vi "medicaoIXV.vi"() -> ()   [LabVIEW 2012]
uses:
  <vilib>/Utility/file.llb/Write To Spreadsheet File (string).vi
  <vilib>/Utility/file.llb/Write To Spreadsheet File (DBL).vi
  <instrlib>/Agilent 6XXX Series/Agilent 6XXX Series.lvlib
panel:
  out "array":dbl[][](array[numeric])
  in  "Tab Control":enum32{"Entrada de dados", "Saída de dados"}(tab)
  out "ON/OFF":bool
  in  "Pontos":dbl
  in  "Tensão máxima":dbl
  in  "Nome da célula":string
  in  "Local":path
  in  "Delay(s)":dbl
  in  "Start":bool
  out "IXV":cluster{"Y":dbl[], "Y":dbl[]}[](graph)
  out "output voltage":dbl
  out "Tensao Atual":dbl
  out "Corrente Atual":dbl
  out "Ponto Atual":i32
  out "TABELA DE DADOS\nTensão(fonte)     Tensão                  Corrente            Pontos":dbl[][](array[numeric]) caption="all rows" format="%0.3f"
  in  "CorrenteGraph":dbl
  in  "error in (no error)":errorcluster
  out "error out":errorcluster
  in  "TensaoGraph":dbl
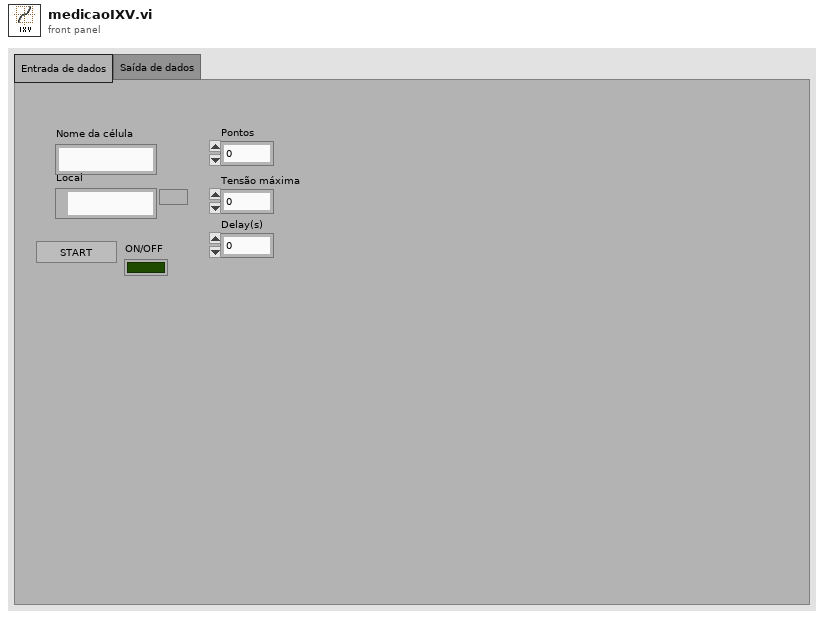
[diagram p1: front panel]
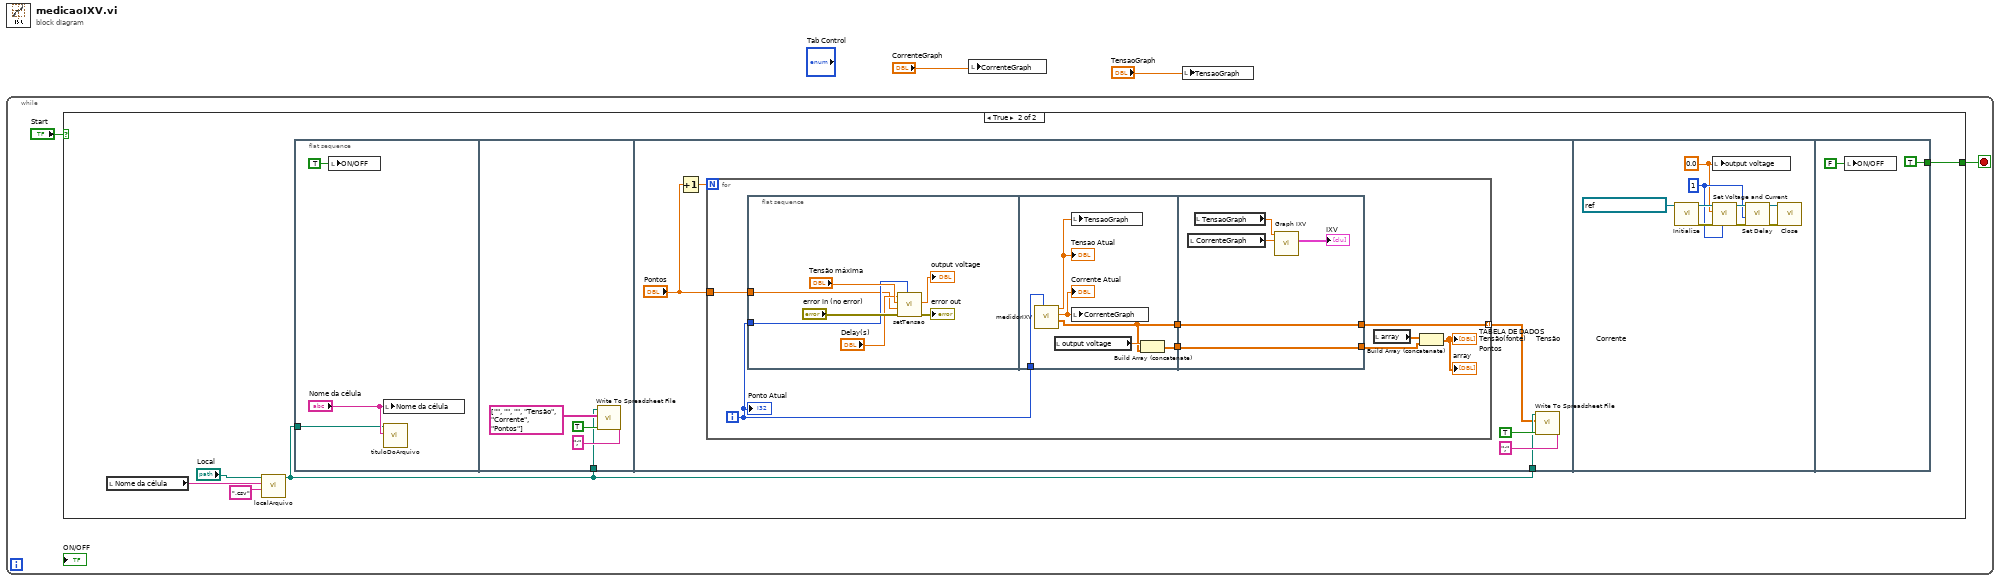
[diagram p0: block diagram]
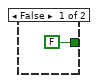
[diagram p2: hidden frame]
diagram:
  n1 = while {
    stop <- w3 stop-if-true
    n2 = case shown="True" "Start" {
      tunnel: [FALSE w10] -> w3
      frame False {
      }
      frame True {
        n3 = local read "Nome da célula"() -> (w6:string)
        n4 = call "localArquivo.vi"("extensão"=".csv", "Nome da célula"=w6, "Local"="Local") -> ("Path"=w8:path)  [unwired: 8 in]
        n5 = flat-sequence {
          tunnel: w8 -> [w12]
          tunnel: w8 -> [w14]
          tunnel: w8 -> [w21]
          tunnel: [TRUE] -> w10
          frame #0 {
            n6 = local write "ON/OFF"(TRUE ("ON/OFF")) -> ()
            n7 = local write "Nome da célula"("Nome da célula") -> ()
            n8 = call "tituloDoArquivo.vi"("Nome da célula"="Nome da célula", "file path (dialog if empty)"=w12) -> ()  [unwired: 10 in]
          }
          frame #1 {
            n9 = call-poly <vilib>:"Write To Spreadsheet File.vi"("delimiter (\\t)"=";" ("delimiter (\\t)"), "append to file? (new file:F)"=TRUE, "2D data"=string[][] [["", "", ""], ["Tensão", "Corrente", "Pontos"]], "file path (dialog if empty)"=w14) -> ()  [unwired: 4 in, 1 out]
          }
          frame #2 {
            n10 = Increment(x="Pontos") -> (x+1=w20:dbl)
            n11 = for {
              N: w20 -> [_]
              tunnel: [w29] -> w18 mode=indexing
              tunnel: "Pontos" -> [w31]
              i -> [w30]
              n12 = flat-sequence {
                tunnel: w31 -> [w34]
                tunnel: w30 -> [w35]
                tunnel: w30 -> [w44]
                tunnel: [w39] -> w28
                tunnel: [w41] -> w27
                tunnel: [w48] -> w26
                tunnel: [w49] -> w29
                tunnel: w28 -> [w49]
                tunnel: w27 -> [w48]
                frame #0 {
                  n13 = call "setTensao.vi"("Ponto"=w35, "error in (no error)"="error in (no error)", "Pontos"=w34, "Tensão máxima"="Tensão máxima", "delay(s)"="Delay(s)") -> ("error out"=→"error out":errorcluster, "output voltage"=→"output voltage":dbl)  [unwired: 5 in]
                }
                frame #1 {
                  n14 = call "medidorIXV.vi"("Ponto"=w44) -> ("Array"=w39:dbl[], "Corrente Atual"=w43:dbl, "Tensao Atual"=w42:dbl)  [unwired: 8 in]
                  "Corrente Atual" <- w43
                  "Tensao Atual" <- w42
                  n15 = local read "output voltage"() -> (w40:dbl)
                  n16 = local write "TensaoGraph"(w42) -> ()
                  n17 = local write "CorrenteGraph"(w43) -> ()
                  n18 = Build Array (concatenate)(w40, w39) -> (w41:dbl[])
                }
                frame #2 {
                  n19 = local read "CorrenteGraph"() -> (w45:dbl)
                  n20 = local read "TensaoGraph"() -> (w46:dbl)
                  n21 = call "Graph IXV"("Y Input"=w45, "X Input"=w46) -> ("XY Graph"=→"IXV":cluster{"Y":dbl[], "Y":dbl[]}[])  [unwired: 3 in, 6 out]
                }
              }
              n22 = local read "array"() -> (w25:dbl[][])
              n23 = Build Array (concatenate)(w25, w26) -> (→"TABELA DE DADOS\nTensão(fonte)     Tensão                  Corrente            Pontos" →"array":dbl[][])
              "Ponto Atual" <- w30
            }
            n24 = call-poly <vilib>:"Write To Spreadsheet File.vi"("delimiter (\\t)"=";" ("delimiter (\\t)"), "append to file? (new file:F)"=TRUE, "2D data"=w18, "file path (dialog if empty)"=w21) -> ()  [unwired: 4 in, 1 out]
          }
          frame #3 {
            w50 = 0.0 ("voltage (0 V)")
            w53 = u8 1 ("channel (1)")
            n25 = call <instrlib>:"Initialize.vi"("VISA resource name"=refnum<visa-resource-name> "GPIB0::5::INSTR") -> ("error out"=w55:errorcluster, "VISA resource name out"=w54:refnum<visa-resource-name>)  [unwired: 9 in]
            n26 = local write "output voltage"(w50) -> ()
            n27 = call <instrlib>:"Set Voltage and Current.vi"("channel (1)"=w53, "error in (no error)"=w55, "voltage (0 V)"=w50, "VISA resource name"=w54) -> ("error out"=w56:errorcluster, "VISA resource name out"=w57:refnum<visa-resource-name>)  [unwired: 6 in]
            n28 = call <instrlib>:"Set Delay.vi"("error in (no error)"=w56, "channel (1)"=w53, "VISA resource name"=w57) -> ("error out"=w51:errorcluster, "VISA resource name out"=w52:refnum<visa-resource-name>)  [unwired: 7 in]
            n29 = call <instrlib>:"Close.vi"("error in (no error)"=w51, "VISA resource name"=w52) -> ()  [unwired: 9 in, 1 out]
          }
          frame #4 {
            n30 = local write "ON/OFF"(FALSE) -> ()
          }
        }
      }
    }
  }
  n31 = local write "CorrenteGraph"("CorrenteGraph") -> ()
  n32 = local write "TensaoGraph"("TensaoGraph") -> ()
